vi "Agilent 34970 JKI Measure Voltage Temperature AJ Version.vi"() -> ()   [LabVIEW 2018]
uses:
  Agilent 34970.lvlib
panel:
  in  "Data Output":string
  out "Temp Output Array":string[](array[string])
  out "Voltage Output Array":string[](array[string])
  in  "Voltage Reading":string
  in  "Temperature Reading":string
  in  "scan rate":i32
  in  "Temperature Channel List":string
  in  "Path":path
  in  "Voltage Channel List":string
  in  "VISA resource name":refnum<visa-resource-name>
  in  "EXIT":bool
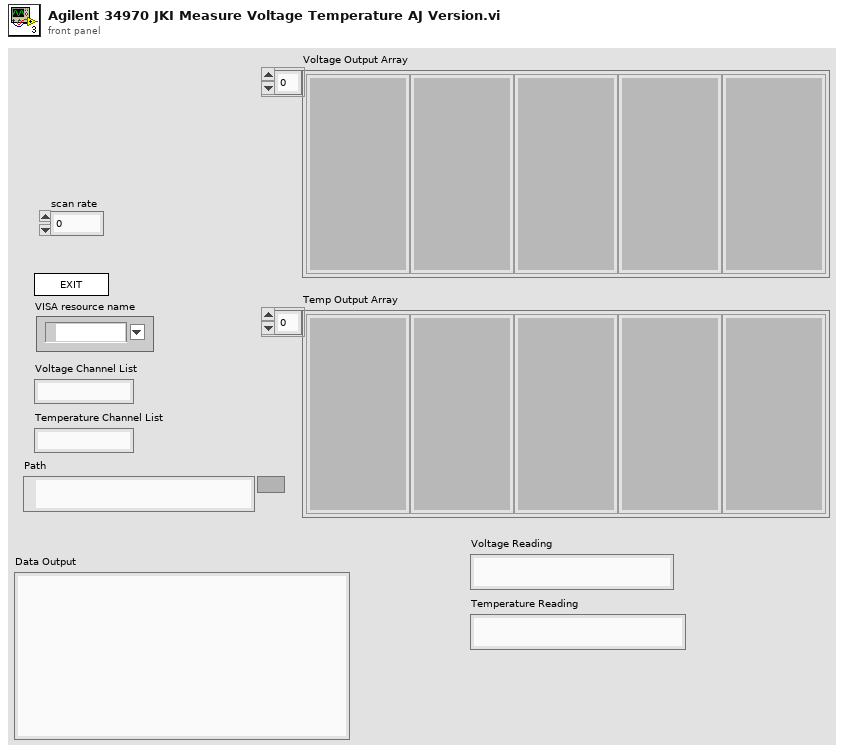
[diagram p1: front panel]
types:
  T1 = enum32{"invalid app kind", "Development System", "Run Time System", "Student Edition", "Embedded LabVIEW", "Evaluation", "Custom"}
  T2 = enum32{"Invalid", "Standard", "Closed", "Hidden", "Minimized", "Maximized"}
  T3 = enum16{"Enable Register", "Event Register", "Operation Complete Bit"}
  T4 = enum16{"Manual", "Minimum", "Maximum", "Infinity"}
  T5 = enum16{"Bus", "Immediate", "External", "Alarm 1", "Alarm 2", "Alarm 3", "Alarm 4", "Timer"}
  T6 = enum16{"100 mV", "1 V", "10 V", "100 V", "300 V", "Minimum", "Maximum"}
  T7 = cluster{"Core":cluster{"Current VI Reference":refnum<vi>, "Close Panel on Exit?":bool}, "VISA resource name":refnum<visa-resource-name>, "Voltage Channel List":string, "Temperature Channel List":string, "Path":path, "Voltage Reading":string, "Temperature Reading":string, "Data Output":string}
  T8 = cluster{"Current VI Reference":refnum<vi>, "Close Panel on Exit?":bool}
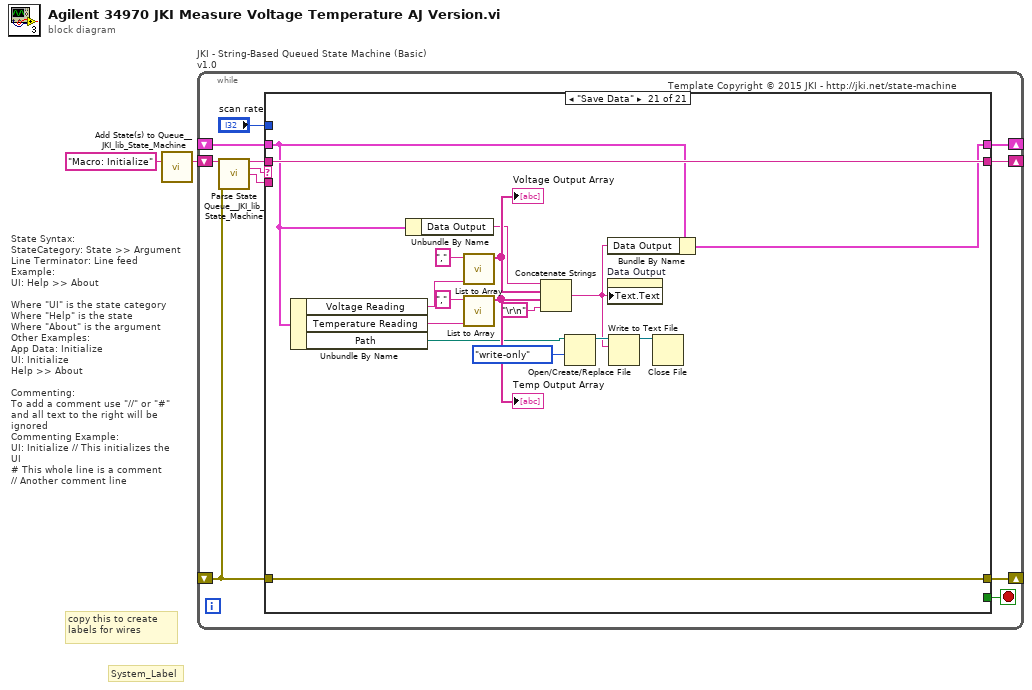
[diagram p0: block diagram]
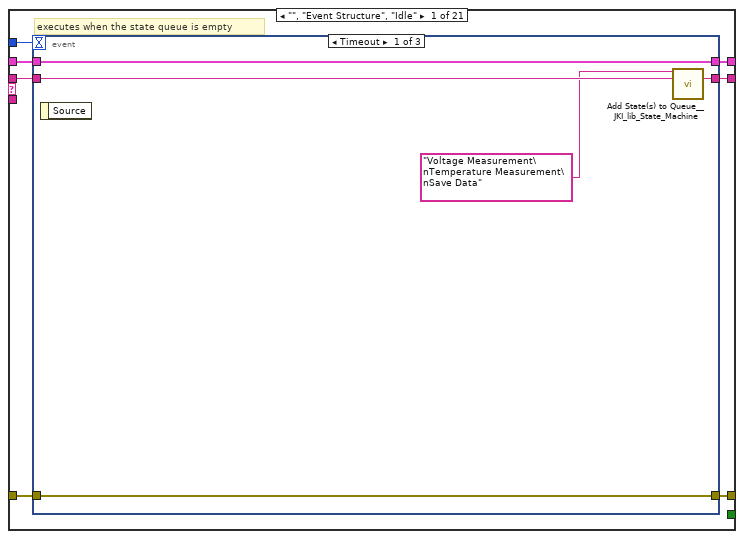
[diagram p2: hidden frame]
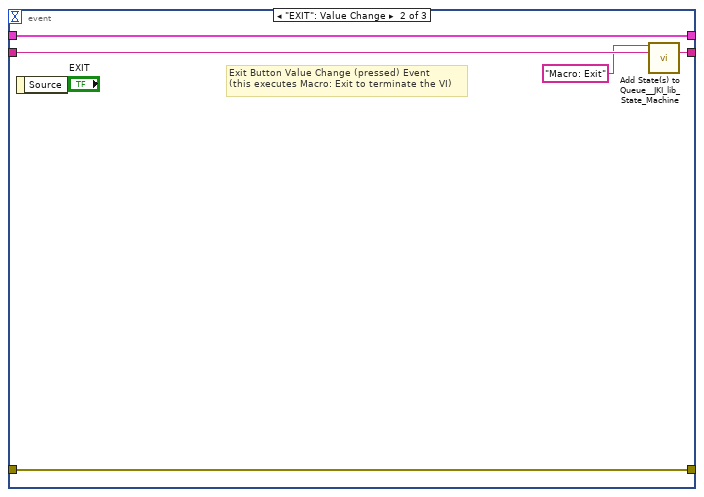
[diagram p3: hidden frame]
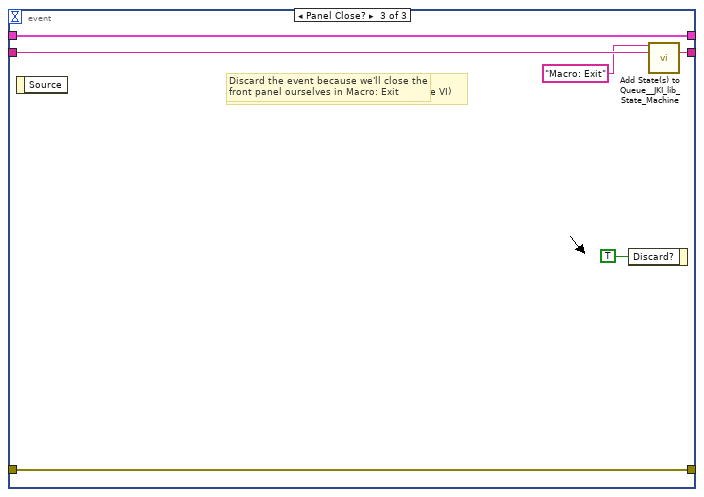
[diagram p4: hidden frame]
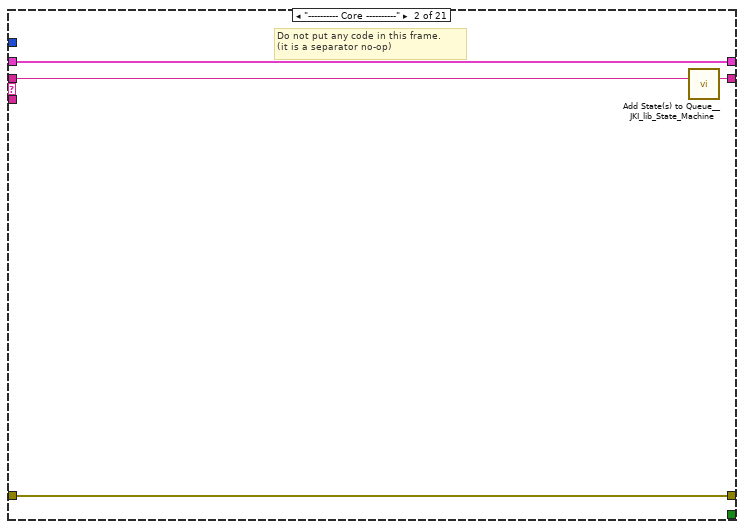
[diagram p5: hidden frame]
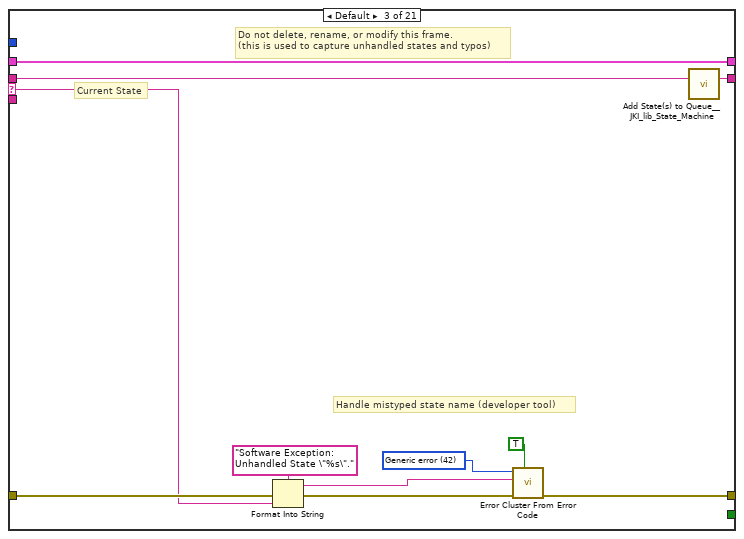
[diagram p6: hidden frame]
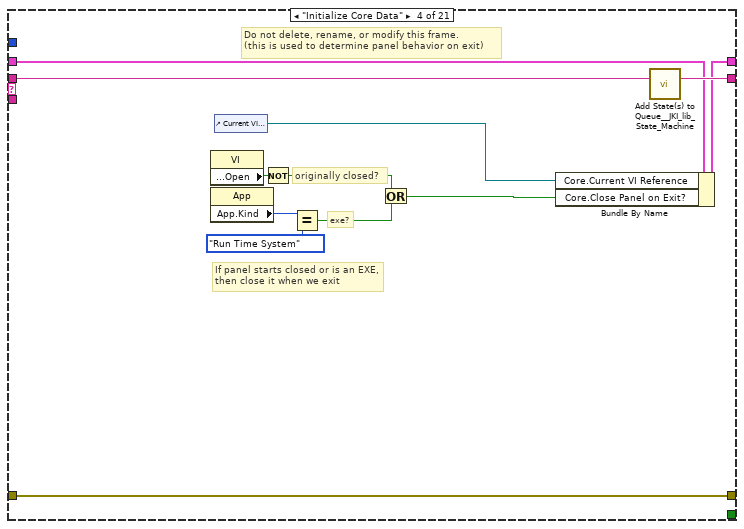
[diagram p7: hidden frame]
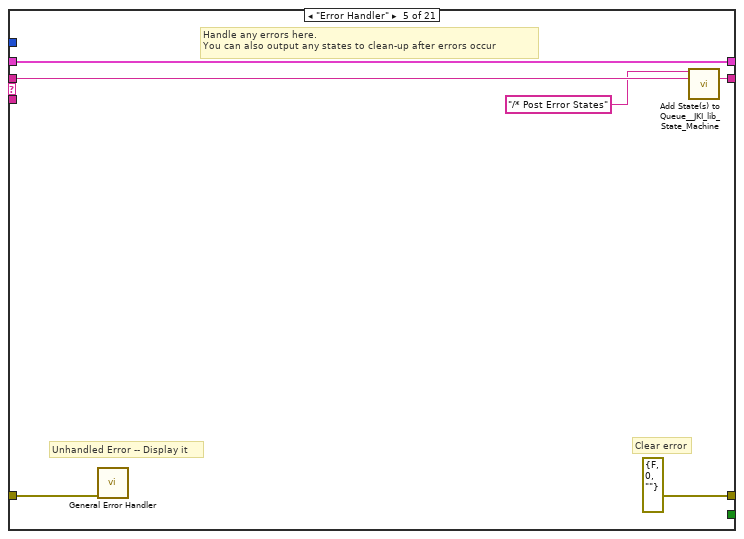
[diagram p8: hidden frame]
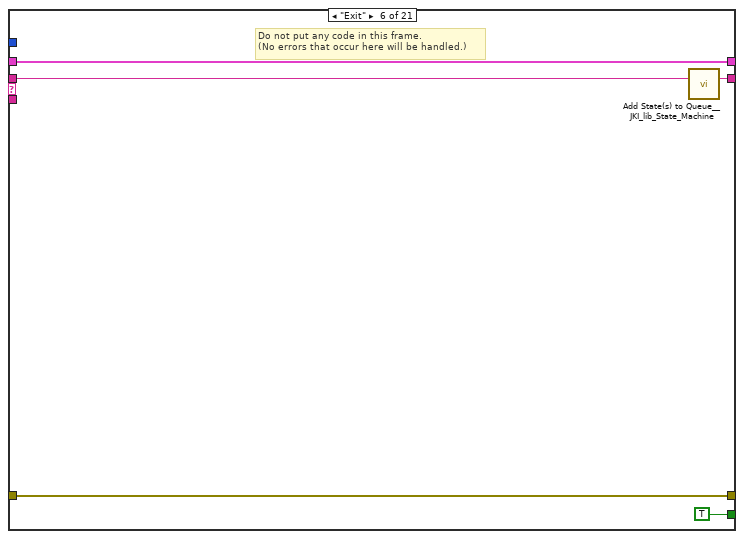
[diagram p9: hidden frame]
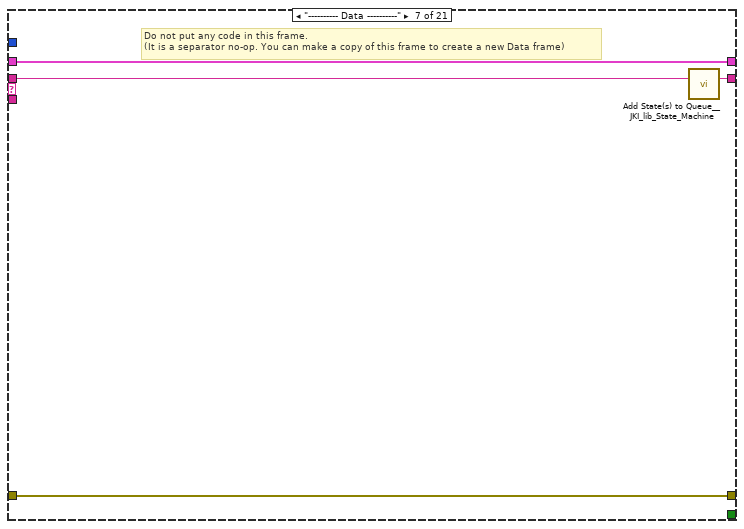
[diagram p10: hidden frame]
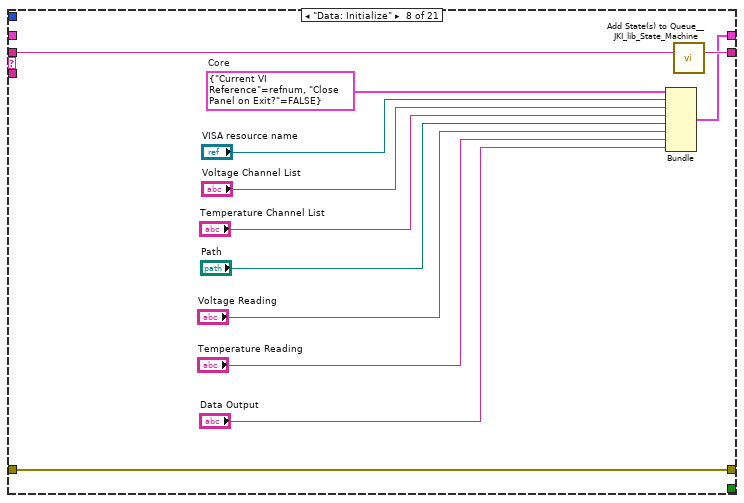
[diagram p11: hidden frame]
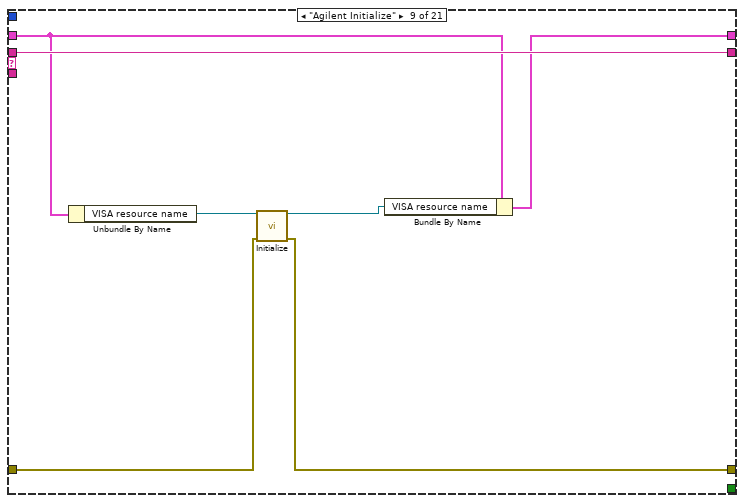
[diagram p12: hidden frame]
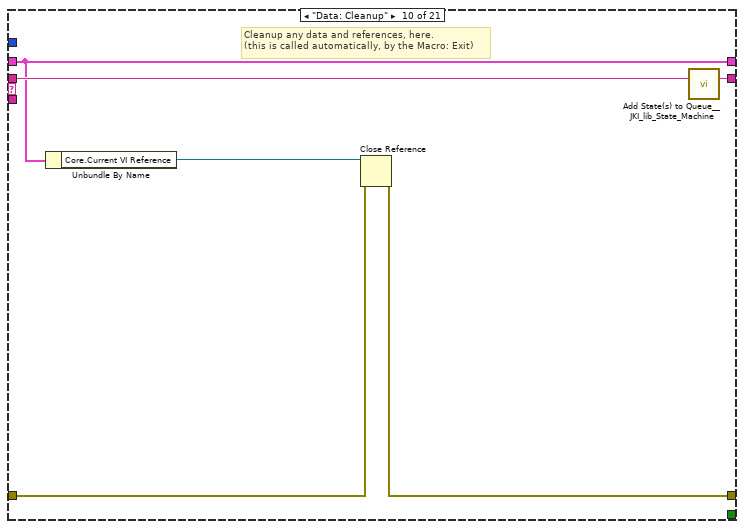
[diagram p13: hidden frame]
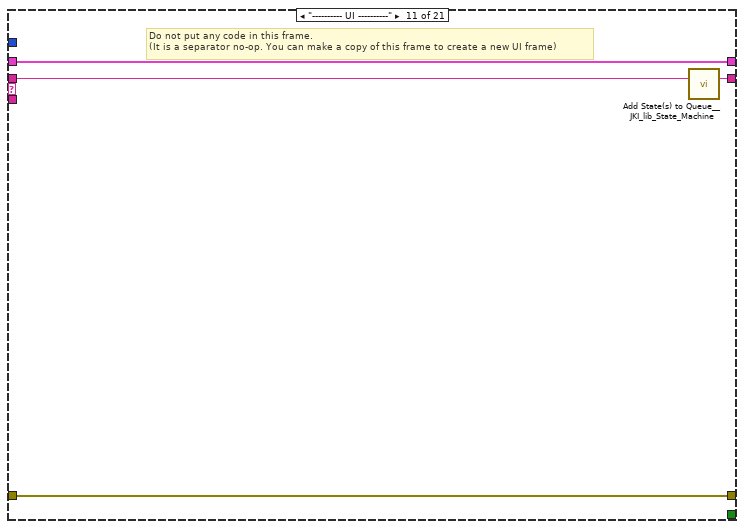
[diagram p14: hidden frame]
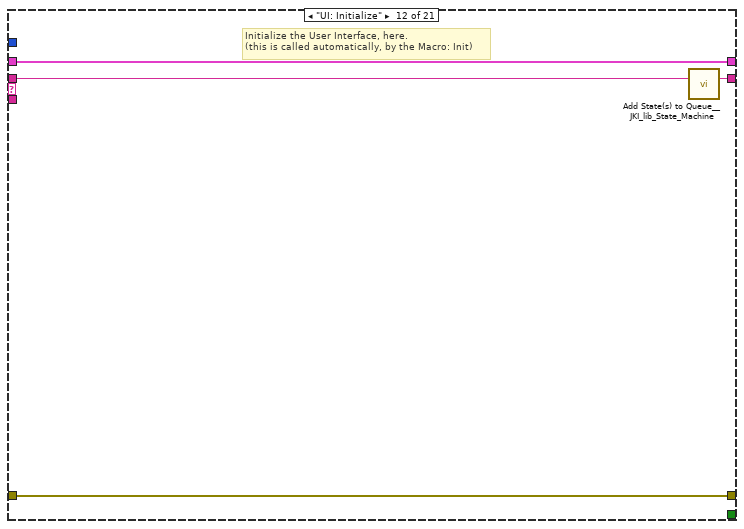
[diagram p15: hidden frame]
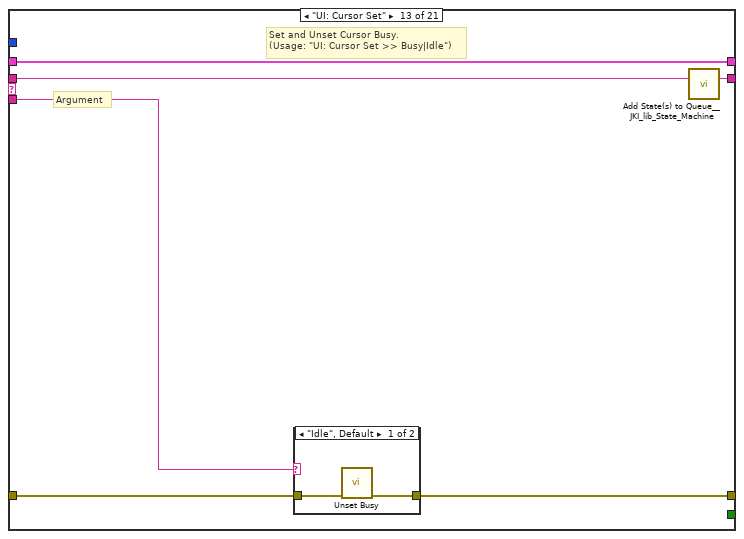
[diagram p16: hidden frame]
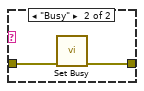
[diagram p17: hidden frame]
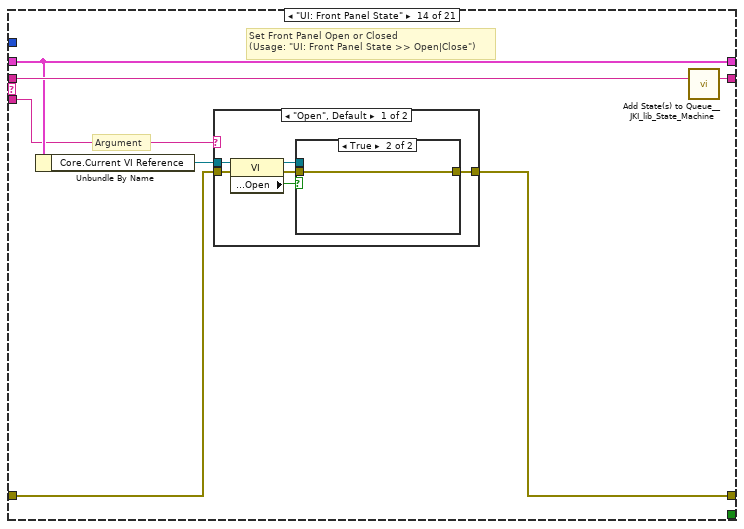
[diagram p18: hidden frame]
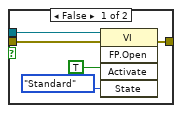
[diagram p19: hidden frame]
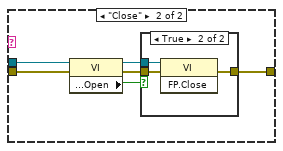
[diagram p20: hidden frame]
diagram:
  # "State Syntax:\nStateCategory: State >> Argument\nLine Terminator: Line feed\nExample:\nUI: Help >> About\n\nWhere \"UI\" is the state category\nWhere \"Help\" is the state\nWhere \"About\" is the argument\nOther Examples:\nApp Data: Initialize\nUI: Initialize\nHelp >> About\n\nCommenting:\nTo add a comment use \"//\" or \"#\" and all text to the right will be ignored\nCommenting Example:\nUI: Initialize // This initializes the UI\n# This whole line is a comment\n// Another comment line"
  # "copy this to create labels for wires"
  # "System_Label"
  n1 = call <vilib>:"Add State(s) to Queue__JKI_lib_State_Machine.vi"("State(s) in (\"\")"="Macro: Initialize") -> ("States Out"=w2:string)  [unwired: 14 in]
  n2 = while "JKI - String-Based Queued State Machine (Basic) v1.0" {
    shift-right: [w6] -> _
    shift-left: _ -> [w5]
    shift-right: [w9] -> _
    shift-left: _ -> [w4]
    shift-right: [w8] -> _
    shift-left: w2 -> [w10]
    stop <- w7 stop-if-true
    # "Template Copyright © 2015 JKI - http://jki.net/state-machine"
    n3 = call <vilib>:"Parse State Queue__JKI_lib_State_Machine.vi"("State Queue"=w10, "Error In (no error)"=w4) -> ("Remaining States"=w12:string, "Current State"=w13:string, "Arguments"=w11:string)  [unwired: 11 in]
    n4 = case shown="\"Save Data\"" w13 {
      selector: w13 -> [_ _ w41 _ _ _ _ _ _ _ _ _ _ _ _ _ _ _ _ _ _]
      tunnel: w12 -> [w20 w40 w45 w63 w69 w74 w78 w90 w97 w103 w107 w111 w117 w128 w154 w159 w169 w173 w201 w227 w244]
      tunnel: w11 -> [_ _ _ _ _ _ _ _ _ _ _ _ w112 w122 _ _ _ _ _ _ _]
      tunnel: w5 -> [w18 w37 w43 w54 w66 w72 w75 _ w93 w98 w104 w109 w115 w124 w151 w156 w166 w170 w176 w203 w229]
      tunnel: [w17 w38 w47 w60 errorcluster {"status"=FALSE, "code"=0, "source"=""} ("error out") w71 w76 w87 w94 w99 w105 w108 w113 w125 w152 w157 w167 w171 w177 w205 w243] -> w9
      tunnel: w4 -> [w16 w38 w46 w60 w65 w71 w76 w87 w95 w100 w105 w108 w114 w126 w152 w157 w167 w171 w198 w207 w243]
      tunnel: [w19 w39 w44 w62 w68 w73 w77 w89 w97 w102 w106 w110 w116 w127 w153 w158 w168 w172 w200 w226 w244] -> w8
      tunnel: [_ _ _ _ _ TRUE _ _ _ _ _ _ _ _ _ _ _ _ _ _ _] -> w7
      tunnel: [w15 w37 w43 w61 w66 w72 w75 w88 w92 w98 w104 w109 w115 w124 w151 w156 w166 w170 w174 w202 w228] -> w6
      tunnel: "scan rate" -> [w14 _ _ _ _ _ _ _ _ _ _ _ _ _ _ _ _ _ _ _ _]
      frame "", "Event Structure", "Idle" {
        # "executes when the state queue is empty"
        n5 = event shown="[0] Timeout" {
          selector: _ -> [_ _ _]
          dyn-events: _ -> [_ _ _]
          timeout: w14 -> [_ _ _]
          tunnel: w20 -> [w25 w30 w36]
          tunnel: [w24 w29 w35] -> w19
          tunnel: w18 -> [w22 w27 w33]
          tunnel: [w23 w28 w34] -> w17
          tunnel: w16 -> [w23 w28 w34]
          tunnel: [w22 w27 w33] -> w15
          event Timeout {
            n6 = event-data() -> ()  [unwired: 1 in, 1 out]
            n7 = call <vilib>:"Add State(s) to Queue__JKI_lib_State_Machine.vi"("State(s) in Front (\"\")"="Voltage Measurement\nTemperature Measurement\nSave Data", "State(s) in (\"\")"=w25) -> ("States Out"=w24:string)  [unwired: 13 in]
          }
          event "EXIT": Value Change {
            # "Exit Button Value Change (pressed) Event\n(this executes Macro: Exit to terminate the VI)"
            n8 = event-data() -> ()  [unwired: 1 in, 1 out]
            n9 = call <vilib>:"Add State(s) to Queue__JKI_lib_State_Machine.vi"("State(s) in Front (\"\")"="Macro: Exit", "State(s) in (\"\")"=w30) -> ("States Out"=w29:string)  [unwired: 13 in]
          }
          event Panel Close? {
            # "Discard the event because we'll close the front panel ourselves in Macro: Exit"
            # "Close Panel button (pressed) Event\n(this executes Macro: Exit to terminate the VI)"
            n10 = event-data() -> ()  [unwired: 1 in, 1 out]
            n11 = event-data("Discard?"=TRUE) -> ()  [unwired: 1 in, 1 out]
            n12 = call <vilib>:"Add State(s) to Queue__JKI_lib_State_Machine.vi"("State(s) in Front (\"\")"="Macro: Exit", "State(s) in (\"\")"=w36) -> ("States Out"=w35:string)  [unwired: 13 in]
          }
        }
      }
      frame "---------- Core ----------" {
        # "Do not put any code in this frame.\n(it is a separator no-op)"
        n13 = call <vilib>:"Add State(s) to Queue__JKI_lib_State_Machine.vi"("State(s) in (\"\")"=w40) -> ("States Out"=w39:string)  [unwired: 14 in]
      }
      frame Default {
        w50 = 42 items=["No error", "Argument error", "Memory is full", "Out of zone", "End of file", "File already open", "Generic file I/O error", "File not found", "File permission error", "Disk is full", "Duplicate path", "Too many files open", "System feature not enabled", "Resource file not found", "Cannot add resource", "Resource not found", "Image not found", "Image memory error", "Pen does not exist", "Config type invalid", "Config token not found", "Config parse error", "Config memory error", "Bad external code format", "Bad external code offset", "External code not present", "Null window", "Destroy window error", "Null menu", "Print aborted", "Bad print record", "Print driver error", "Windows error during printing", "Memory error during printing", "Print dialog error", "Generic print error", "Invalid device refnum", "Device not found", "Device parameter error", "Device unit error", "Cannot open device", "Device call aborted", "Generic error", "Cancelled by user", "Object ID too low", "Object ID too high", "Object not in heap", "Unknown heap", "Unknown object (invalid DefProc)", "Unknown object (DefProc not in table)", "Message out of range", "Invalid (null) method", "Unknown message", "Manager call not supported", "Bad address", "Network operation in progress", "Network operation timed out", "Connection is busy", "Network attribute not supported", "Network error", "Address in use", "System out of memory", "Connection aborted", "Connection refused", "Not connected", "Already connected", "Connection closed", "Initialization error (interapplication manager)", "Bad occurrence", "Wait on unbound occurrence handler", "Occurrence queue overflow", "Datalog type conflict", "Unused", "Unrecognized type (interapplication manager)", "Memory corrupt", "Failed to make temporary DLL", "Old CIN version", "Drag socket not found", "Failed to load drop-object", "Failed to register OLE object", "Failed to release OLE object", "Format specifier type mismatch", "Unknown format specifier", "Too few format specifiers", "Too many format specifiers", "Scan failed", "Newer CIN version", "Error converting to variant", "Runtime menu error", "Password tampered", "Variant attribute not found", "Incompatible variant data type", "Event data is not available", "Event Store is not present", "Occurrence is not found", "Event Queue is not created", "Event info is not available", "Refnum passed is NULL", "Error retrieving Class GUID", "Error retrieving CoClass GUID", "Error retrieving TypeLib GUID.", "Bad built application magic bytes.", "Specific driver is different from the specific driver associated with the Logical Name.", "There is no session opened to the class driver.", "Max Error", "MAX - Error with config objects", "MAX - Error loading configuration", "MAX - Group not supported"]
        # "Current State"
        # "Do not delete, rename, or modify this frame.\n(this is used to capture unhandled states and typos)"
        # "Handle mistyped state name (developer tool)"
        n14 = Format Into String(format string="Software Exception: Unhandled State \"%s\"." ("message"), error in=w46, w41) -> (resulting string=w49:string, error out=w48:errorcluster)  [unwired: 1 in]
        n15 = call <vilib>:"Error Cluster From Error Code.vi"("show call chain? (False)"=TRUE, "error in (no error)"=w48, "error message (\"\")"=w49, "error code (0)"=w50) -> ("error out"=w47:errorcluster)  [unwired: 5 in]
        n16 = call <vilib>:"Add State(s) to Queue__JKI_lib_State_Machine.vi"("State(s) in (\"\")"=w45) -> ("States Out"=w44:string)  [unwired: 14 in]
      }
      frame "Initialize Core Data" {
        # "Do not delete, rename, or modify this frame.\n(this is used to determine panel behavior on exit)"
        # "originally closed?"
        # "exe?"
        # "If panel starts closed or is an EXE, then close it when we exit"
        n17 = property class="VI"() -> ("Front Panel.Open"=w59:bool)  [unwired: 2 in, 2 out]
        n18 = property class="App"() -> ("App.Kind"=w58:T1)  [unwired: 2 in, 2 out]
        n19 = control-ref of="Current VI Reference"() -> (w52:refnum<vi>)
        n20 = Not(x=w59) -> (.not. x?=w56:bool)
        n21 = Equal?(x=w58, y=T1."Run Time System" ("Application:Kind")) -> (x = y?=w55:bool)
        n22 = Or(x=w56, y=w55) -> (x .or. y?=w53:bool)
        n23 = Bundle By Name(cluster=w54, "Core.Current VI Reference"=w52, "Core.Close Panel on Exit?"=w53) -> (w61:T7)
        n24 = call <vilib>:"Add State(s) to Queue__JKI_lib_State_Machine.vi"("State(s) in (\"\")"=w63) -> ("States Out"=w62:string)  [unwired: 14 in]
      }
      frame "Error Handler" {
        # "Unhandled Error -- Display it"
        # "Handle any errors here.\nYou can also output any states to clean-up after errors occur"
        # "Clear error"
        n25 = call <vilib>:"General Error Handler.vi"("error in (no error)"=w65) -> ()  [unwired: 10 in, 5 out]
        n26 = call <vilib>:"Add State(s) to Queue__JKI_lib_State_Machine.vi"("State(s) in Front (\"\")"="/* Post Error States", "State(s) in (\"\")"=w69) -> ("States Out"=w68:string)  [unwired: 13 in]
      }
      frame "Exit" {
        # "Do not put any code in this frame.\n(No errors that occur here will be handled.)"
        n27 = call <vilib>:"Add State(s) to Queue__JKI_lib_State_Machine.vi"("State(s) in (\"\")"=w74) -> ("States Out"=w73:string)  [unwired: 14 in]
      }
      frame "---------- Data ----------" {
        # "Do not put any code in this frame.\n(It is a separator no-op. You can make a copy of this frame to create a new Data frame)"
        n28 = call <vilib>:"Add State(s) to Queue__JKI_lib_State_Machine.vi"("State(s) in (\"\")"=w78) -> ("States Out"=w77:string)  [unwired: 14 in]
      }
      frame "Data: Initialize" {
        w86 = T8 {"Current VI Reference"=refnum, "Close Panel on Exit?"=FALSE}  # Core
        n29 = Bundle("Core"=w86, "VISA resource name"="VISA resource name", "Voltage Channel List"="Voltage Channel List", "Temperature Channel List"="Temperature Channel List", "Path"="Path", "Voltage Reading"="Voltage Reading", "Temperature Reading"="Temperature Reading", "Data Output"="Data Output") -> (w88:T7)  [unwired: 1 in]
        n30 = call <vilib>:"Add State(s) to Queue__JKI_lib_State_Machine.vi"("State(s) in (\"\")"=w90) -> ("States Out"=w89:string)  [unwired: 14 in]
      }
      frame "Agilent Initialize" {
        n31 = Unbundle By Name(w93) -> ("VISA resource name"=w96:refnum<visa-resource-name>)
        n32 = call "Initialize.vi"("VISA Resource Name"=w96, "error in (no error)"=w95) -> ("VISA Resource Name Out"=w91:refnum<visa-resource-name>, "error out"=w94:errorcluster)  [unwired: 12 in]
        n33 = Bundle By Name(cluster=w93, "VISA resource name"=w91) -> (w92:T7)
      }
      frame "Data: Cleanup" {
        # "Cleanup any data and references, here.\n(this is called automatically, by the Macro: Exit)"
        n34 = Unbundle By Name(w98) -> ("Core.Current VI Reference"=w101:refnum<vi>)
        n35 = Close Reference(reference=w101, error in (no error)=w100) -> (error out=w99:errorcluster)
        n36 = call <vilib>:"Add State(s) to Queue__JKI_lib_State_Machine.vi"("State(s) in (\"\")"=w103) -> ("States Out"=w102:string)  [unwired: 14 in]
      }
      frame "---------- UI ----------" {
        # "Do not put any code in this frame.\n(It is a separator no-op. You can make a copy of this frame to create a new UI frame)"
        n37 = call <vilib>:"Add State(s) to Queue__JKI_lib_State_Machine.vi"("State(s) in (\"\")"=w107) -> ("States Out"=w106:string)  [unwired: 14 in]
      }
      frame "UI: Initialize" {
        # "Initialize the User Interface, here.\n(this is called automatically, by the Macro: Init)"
        n38 = call <vilib>:"Add State(s) to Queue__JKI_lib_State_Machine.vi"("State(s) in (\"\")"=w111) -> ("States Out"=w110:string)  [unwired: 14 in]
      }
      frame "UI: Cursor Set" {
        # "Argument"
        # "Set and Unset Cursor Busy.\n(Usage: \"UI: Cursor Set >> Busy|Idle\")"
        n39 = case shown="\"Idle\", Default" w112 {
          tunnel: w114 -> [w119 w121]
          tunnel: [w118 w120] -> w113
          frame "Idle", Default {
            n40 = call <vilib>:"Unset Busy.vi"("error in (no error)"=w119) -> ("error out"=w118:errorcluster)  [unwired: 10 in]
          }
          frame "Busy" {
            n41 = call <vilib>:"Set Busy.vi"("error in (no error)"=w121) -> ("error out"=w120:errorcluster)  [unwired: 9 in, 1 out]
          }
        }
        n42 = call <vilib>:"Add State(s) to Queue__JKI_lib_State_Machine.vi"("State(s) in (\"\")"=w117) -> ("States Out"=w116:string)  [unwired: 14 in]
      }
      frame "UI: Front Panel State" {
        # "Argument"
        # "Set Front Panel Open or Closed\n(Usage: \"UI: Front Panel State >> Open|Close\")"
        n43 = Unbundle By Name(w124) -> ("Core.Current VI Reference"=w123:refnum<vi>)
        n44 = case shown="\"Open\", Default" w122 {
          tunnel: w126 -> [w132 w145]
          tunnel: [w134 w146] -> w125
          tunnel: w123 -> [w133 w143]
          frame "Open", Default {
            n45 = property class="VI"(reference=w133, error in=w132) -> (reference out=w130:refnum<vi>, error out=w131:errorcluster, "Front Panel.Open"=w129:bool)
            n46 = case shown="True" w129 {
              tunnel: [w137 w140] -> w134
              tunnel: w131 -> [w136 w140]
              tunnel: w130 -> [w135 _]
              frame False {
                n47 = invoke class="VI" method="FP.Open"(reference=w135, error in=w136, "Activate"=TRUE, "State"=T2."Standard") -> (error out=w137:errorcluster)  [unwired: 1 in, 4 out]
              }
              frame True {
              }
            }
          }
          frame "Close" {
            n48 = property class="VI"(reference=w143, error in=w145) -> (reference out=w142:refnum<vi>, error out=w144:errorcluster, "Front Panel.Open"=w141:bool)
            n49 = case shown="True" w141 {
              tunnel: [w147 w150] -> w146
              tunnel: w144 -> [w147 w149]
              tunnel: w142 -> [_ w148]
              frame False {
              }
              frame True {
                n50 = invoke class="VI" method="FP.Close"(reference=w148, error in=w149) -> (error out=w150:errorcluster)  [unwired: 1 in, 2 out]
              }
            }
          }
        }
        n51 = call <vilib>:"Add State(s) to Queue__JKI_lib_State_Machine.vi"("State(s) in (\"\")"=w128) -> ("States Out"=w127:string)  [unwired: 14 in]
      }
      frame "---------- Macro ----------" {
        # "Do not put any code in this frame.\n(It is a separator no-op. You can make a copy of this frame to create a new Macro frame)"
        n52 = call <vilib>:"Add State(s) to Queue__JKI_lib_State_Machine.vi"("State(s) in (\"\")"=w154) -> ("States Out"=w153:string)  [unwired: 14 in]
      }
      frame "Macro: Initialize" {
        w155 = "Data: Initialize\nInitialize Core Data\nAgilent Initialize\nUI: Initialize\nUI: Front Panel State >> Open"  # Data: Initialize Initialize Core Data Agilent Initialize UI: Initialize UI: Front Panel State >> Open
        # "Initialization Macro\n(This is called once, when the VI starts)"
        n53 = call <vilib>:"Add State(s) to Queue__JKI_lib_State_Machine.vi"("State(s) in Front (\"\")"=w155, "State(s) in (\"\")"=w159) -> ("States Out"=w158:string)  [unwired: 13 in]
      }
      frame "Macro: Exit" {
        # "Exit Macro\n(This is called once, when the VI exits)"
        n54 = Unbundle By Name(w166) -> ("Core.Close Panel on Exit?"=w165:bool)
        n55 = Select(t="UI: Front Panel State >> Close", s=w165, f="") -> (s? t:f=w162:string)
        n56 = call <vilib>:"Add State(s) to Queue__JKI_lib_State_Machine.vi"("State(s) in (\"\")"=w162, "State(s) at Back (\"\")"="Data: Cleanup\nExit") -> ("States Out"=w160:string)  [unwired: 13 in]
        n57 = call <vilib>:"Add State(s) to Queue__JKI_lib_State_Machine.vi"("State(s) in Front (\"\")"=w160, "State(s) in (\"\")"=w169) -> ("States Out"=w168:string)  [unwired: 13 in]
      }
      frame "---------- New Category ----------" {
        # "Template Separator\n(You can make a copy of, or modify, this frame)"
        n58 = call <vilib>:"Add State(s) to Queue__JKI_lib_State_Machine.vi"("State(s) in (\"\")"=w173) -> ("States Out"=w172:string)  [unwired: 14 in]
      }
      frame "Voltage Measurement" {
        n59 = Unbundle By Name(w176) -> ("VISA resource name"=w199:refnum<visa-resource-name>, "Voltage Channel List"=w190:string)
        n60 = call "Conf Voltage.vi"("VISA Resource Name"=w199, "Set/Check (F:Set)"=FALSE, "Autorange? (F:Off)"=FALSE, "Range (6:Max)"=T6."Maximum", "error in (no error)"=w198, "Channel List (empty)"=w190) -> ("VISA Resource Name Out"=w193:refnum<visa-resource-name>, "error out"=w194:errorcluster)  [unwired: 7 in, 1 out]
        n61 = call "Conf Scan List.vi"("Scan List (empty)"=w190, "error in (no error)"=w194, "VISA Resource Name"=w193) -> ("error out"=w191:errorcluster, "VISA Resource Name Out"=w192:refnum<visa-resource-name>)  [unwired: 6 in, 1 out]
        n62 = call "Conf Scan.vi"("VISA Resource Name"=w192, "error in (no error)"=w191, "Channel List (empty)"=w190) -> ("VISA Resource Name Out"=w189:refnum<visa-resource-name>, "error out"=w188:errorcluster)  [unwired: 10 in, 1 out]
        n63 = call "Conf Trigger.vi"("VISA Resource Name"=w189, "Wait for Trigger? (F:No)"=TRUE, "Source (1:Immediate)"=T5."Immediate", "error in (no error)"=w188, "Max Trigger Count (3:Inf)"=T4."Manual") -> ("VISA Resource Name Out"=w184:refnum<visa-resource-name>, "error out"=w183:errorcluster)  [unwired: 8 in, 1 out]
        n64 = call "Standard Event Status.vi"("Set/Check? (F:Set)"=TRUE, "error in (no error)"=w183, "Check Parameter (0:Enable Reg)"=T3."Operation Complete Bit", "VISA Resource Name"=w184) -> ("error out"=w179:errorcluster, "VISA Resource Name Out"=w180:refnum<visa-resource-name>)  [unwired: 5 in, 1 out]
        n65 = call "Read.vi"("error in (no error)"=w179, "# Channels (1)"=2, "VISA Resource Name"=w180) -> ("error out"=w177:errorcluster, "Readings"=w175:string)  [unwired: 5 in, 2 out]
        n66 = Bundle By Name(cluster=w176, "Voltage Reading"=w175) -> (w174:T7)
        n67 = property on="Voltage Reading" class="Str"("Text.Text"=w175) -> ()  [unwired: 2 in, 2 out]
        n68 = call <vilib>:"Add State(s) to Queue__JKI_lib_State_Machine.vi"("State(s) in (\"\")"=w201) -> ("States Out"=w200:string)  [unwired: 14 in]
      }
      frame "Temperature Measurement" {
        n69 = Unbundle By Name(w203) -> ("VISA resource name"=w210:refnum<visa-resource-name>, "Temperature Channel List"=w211:string)
        n70 = call "Conf Temperature.vi"("VISA Resource Name"=w210, "Set/Check? (F:Set)"=FALSE, "error in (no error)"=w207, "Channel List(empty)"=w211) -> ("VISA Resource Name Out"=w209:refnum<visa-resource-name>, "error out"=w208:errorcluster)  [unwired: 9 in, 1 out]
        n71 = call "Conf Scan List.vi"("Scan List (empty)"=w211, "error in (no error)"=w208, "VISA Resource Name"=w209) -> ("error out"=w224:errorcluster, "VISA Resource Name Out"=w225:refnum<visa-resource-name>)  [unwired: 6 in, 1 out]
        n72 = call "Conf Scan.vi"("VISA Resource Name"=w225, "error in (no error)"=w224, "Channel List (empty)"=w211) -> ("VISA Resource Name Out"=w223:refnum<visa-resource-name>, "error out"=w222:errorcluster)  [unwired: 10 in, 1 out]
        n73 = call "Conf Trigger.vi"("VISA Resource Name"=w223, "Wait for Trigger? (F:No)"=TRUE, "Source (1:Immediate)"=T5."Immediate", "error in (no error)"=w222, "Max Trigger Count (3:Inf)"=T4."Manual") -> ("VISA Resource Name Out"=w218:refnum<visa-resource-name>, "error out"=w217:errorcluster)  [unwired: 8 in, 1 out]
        n74 = call "Standard Event Status.vi"("Set/Check? (F:Set)"=TRUE, "error in (no error)"=w217, "Check Parameter (0:Enable Reg)"=T3."Operation Complete Bit", "VISA Resource Name"=w218) -> ("error out"=w213:errorcluster, "VISA Resource Name Out"=w214:refnum<visa-resource-name>)  [unwired: 5 in, 1 out]
        n75 = call "Read.vi"("error in (no error)"=w213, "# Channels (1)"=2, "VISA Resource Name"=w214) -> ("error out"=w205:errorcluster, "Readings"=w204:string)  [unwired: 5 in, 2 out]
        n76 = Bundle By Name(cluster=w203, "Temperature Reading"=w204) -> (w202:T7)
        n77 = property on="Temperature Reading" class="Str"("Text.Text"=w204) -> ()  [unwired: 2 in, 2 out]
        n78 = call <vilib>:"Add State(s) to Queue__JKI_lib_State_Machine.vi"("State(s) in (\"\")"=w227) -> ("States Out"=w226:string)  [unwired: 14 in]
      }
      frame "Save Data" {
        n79 = Unbundle By Name(w229) -> ("Voltage Reading"=w240:string, "Temperature Reading"=w239:string, "Path"=w234:path)
        n80 = Unbundle By Name(w229) -> ("Data Output"=w231:string)
        n81 = call "List to Array.vi"("List (empty)"=w240, "Separator (,)"=",") -> ("Output String Array"=w237:string[])  [unwired: 8 in, 1 out]
        "Voltage Output Array" <- w237
        n82 = call "List to Array.vi"("List (empty)"=w239, "Separator (,)"=",") -> ("Output String Array"=w238:string[])  [unwired: 8 in, 1 out]
        "Temp Output Array" <- w238
        n83 = Concatenate Strings(w231, w237, w238, "\r\n") -> (w230:string)
        n84 = Open/Create/Replace File(file path (use dialog)=w234, access (0:read/write)=enum16{"read/write", "read-only", "write-only"}."write-only") -> (refnum out=w236:refnum<file>)  [unwired: 4 in, 2 out]
        n85 = Bundle By Name(cluster=w229, "Data Output"=w230) -> (w228:T7)
        n86 = property on="Data Output" class="Str"("Text.Text"=w230) -> ()  [unwired: 2 in, 2 out]
        n87 = Write to Text File(file (use dialog)=w236, text=w230) -> (refnum out=w235:refnum<file>)  [unwired: 2 in, 2 out]
        n88 = Close File(refnum=w235) -> ()  [unwired: 1 in, 2 out]
      }
    }
  }
